vi "CalculateOdometry.vi"(5 "Left Wheel Distance":dbl, 6 "Right Wheel Distance":dbl, 7 "Wheel Base":dbl) -> (0 "Distance":dbl, 1 "theta":dbl, 2 "X":dbl, 3 "Y":dbl, 4 "Heading":dbl)   [LabVIEW 2015]
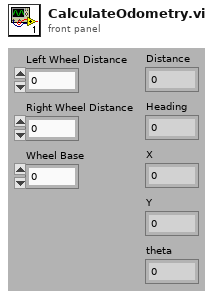
[diagram p1: front panel]
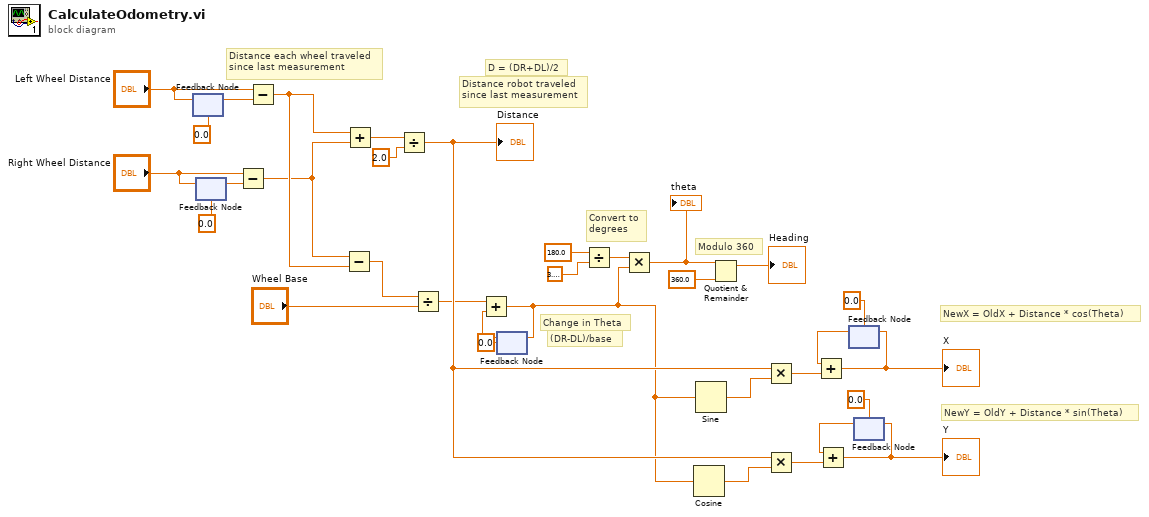
[diagram p0: block diagram]
diagram:
  # "NewY = OldY + Distance * sin(Theta)"
  # "NewX = OldX + Distance * cos(Theta)"
  # "(DR-DL)/base"
  # "D = (DR+DL)/2"
  # "Distance robot traveled\nsince last measurement"
  # "Distance each wheel traveled\nsince last measurement"
  # "Modulo 360"
  # "Convert to\ndegrees"
  # "Change in Theta"
  n1 = feedback-in #1("Left Wheel Distance") -> ()
  n2 = feedback #1(0.0 ("Left Wheel Distance")) -> (w18:dbl)
  n3 = feedback-in #2("Right Wheel Distance") -> ()
  n4 = feedback #2(0.0 ("Right Wheel Distance")) -> (w15:dbl)
  n5 = Subtract(x="Right Wheel Distance", y=w15) -> (x-y=w13:dbl)
  n6 = Subtract(x="Left Wheel Distance", y=w18) -> (x-y=w16:dbl)
  n7 = Subtract(x=w13, y=w16) -> (x-y=w21:dbl)
  n8 = Add(x=w16, y=w13) -> (x+y=w19:dbl)
  n9 = Divide(x=w19, y=2.0) -> (x/y=w27:dbl)
  "Distance" <- w27
  n10 = Divide(x=w21, y="Wheel Base") -> (x/y=w1:dbl)
  n11 = feedback #3(0.0 ("Left Wheel Distance")) -> (w2:dbl)
  n12 = Add(x=w1, y=w2) -> (x+y=w3:dbl)
  n13 = feedback-in #3(w3) -> ()
  n14 = Divide(x=180.0, y=3.141592653589793) -> (x/y=w30:dbl)
  n15 = Multiply(x=w30, y=w3) -> (x*y=w32:dbl)
  "theta" <- w32
  n16 = Cosine(x=w3) -> (cos(x)=w26:dbl)
  n17 = Sine(x=w3) -> (sin(x)=w25:dbl)
  n18 = Quotient & Remainder(x=w32, y=360.0) -> (x-y*floor(x/y)=→"Heading":dbl)  [unwired: 1 out]
  n19 = Multiply(x=w27, y=w25) -> (x*y=w24:dbl)
  n20 = Multiply(x=w27, y=w26) -> (x*y=w23:dbl)
  n21 = feedback #4(0.0 ("Left Wheel Distance")) -> (w8:dbl)
  n22 = Add(x=w8, y=w24) -> (x+y=w9:dbl)
  "X" <- w9
  n23 = feedback-in #4(w9) -> ()
  n24 = feedback #5(0.0 ("Left Wheel Distance")) -> (w5:dbl)
  n25 = Add(x=w5, y=w23) -> (x+y=w6:dbl)
  "Y" <- w6
  n26 = feedback-in #5(w6) -> ()
